vi "Teleop.vi"(0 "Call Context":T3=enum."Stop", 1 "Match Info":T2={"Autonomous Elapsed Seconds"=7.637, "TeleOp Elapsed Seconds"=2.279, "Disabled Elapsed Seconds"=0.688, "Visited Autonomous"=TRUE, "Visited TeleOp"=TRUE, "Visited Disabled"=TRUE, "Autonomous Settings"={"Autonomous Style"=enum."Independent", "VI Refnum"=refnum}}) -> ()   [LabVIEW 2018]
doc: "This VI is called for each TeleOp packet received from the DS where the robot is not disabled. It is often used to read from the joysticks and update I/O or to update setpoints for timed control loops. It should complete and return within 20 milliseconds or it may miss DS packets."
uses:
  <vilib>/Rock Robotics/WPI/DriverStation/WPI_DriverStationDerivedRobotMode.ctl
  <vilib>/Rock Robotics/WPI/DriverStation/WPI_DriverStationMatch Info.ctl
  <vilib>/Rock Robotics/WPI/ThirdParty/Phoenix-LabVIEW/Motor Controller/Controls/CTRE_Phoenix_MotorControl_MotionProfileTrajectoryPoint.ctl
  Subsystems/HatchPanel/hatchPanelNotifierCluster.ctl
  Subsystems/HatchPanel/hatchPanelEnum.ctl
  Subsystems/Cargo/cargoNotifier.ctl
  Subsystems/Cargo/cargoEnum.ctl
  Subsystems/LineAlignment/LineAlignNotifier.ctl
  Subsystems/Drive/gear notifier.ctl
  Subsystems/Climb/climbStateEnum.ctl
  Subsystems/Drive/driveCommandEnum.ctl
  Subsystems/Sensors/Limelight/LimelightPipelineMode.ctl
  Subsystems/Sensors/Limelight/LimelightModeEnum.ctl
  Subsystems/Drive/MotionProfile/Constants.vi
  <vilib>/Rock Robotics/WPI/ThirdParty/Phoenix-LabVIEW/Pigeon IMU/CTRE_PigeonIMU_TareType.ctl
panel:
  out "Output Path Points":T1[](array[typedef])
  in  "Pathname":string="L1LeftToLRF"
  # "hi there"
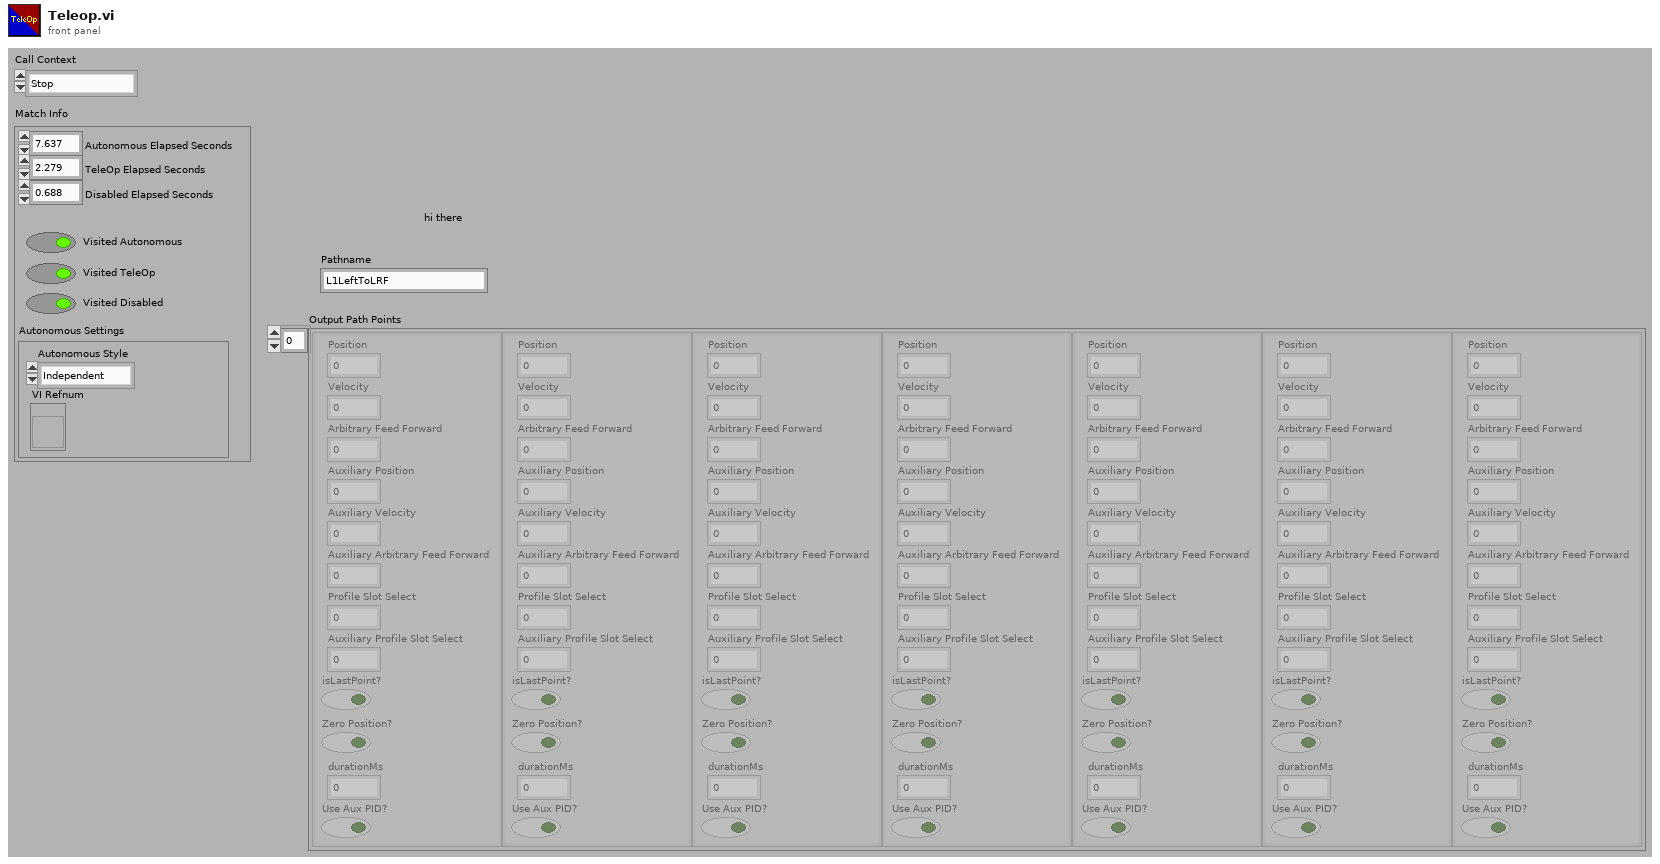
[diagram p1: front panel]
types:
  T1 = typedef "CTRE_Phoenix_MotorControl_MotionProfileTrajectoryPoint.ctl" = cluster{"Position":dbl, "Velocity":dbl, "Arbitrary Feed Forward":dbl, "Auxiliary Position":dbl, "Auxiliary Velocity":dbl, "Auxiliary Arbitrary Feed Forward":dbl, "Profile Slot Select":i32, "Auxiliary Profile Slot Select":i32, "isLastPoint?":bool, "Zero Position?":bool, "durationMs":u32, "Use Aux PID?":bool}
  T2 = typedef "WPI_DriverStationMatch Info.ctl" = cluster{"Autonomous Elapsed Seconds":dbl, "TeleOp Elapsed Seconds":dbl, "Disabled Elapsed Seconds":dbl, "Visited Autonomous":bool, "Visited TeleOp":bool, "Visited Disabled":bool, "Autonomous Settings":cluster{"Autonomous Style":enum16{"Iterative", "Independent"}, "VI Refnum":refnum<vi>}}
  T3 = typedef "WPI_DriverStationDerivedRobotMode.ctl" = enum16{"Init", "Execute", "Stop"}
  T4 = enum16{"Stach Open to Gather", "Stach Wait for Gather Extend", "Stach Gather Extended", "Stach Wait for Grab Panel", "Stach Grab Panel", "Stach Closed to Score", "Stach Wait for Sonar Signal", "Stach Wait for Score Extend", "Stach Ready to Score ", "Stach Wait for Release Panel", "Stach Release Panel", "Stach Wait for Gather Retract", "Stach Wait for Score Retract", "Stach Wait for Gather Unlock", "Stach Wait for Score Unlock", "Stach Gather End Lock", "Stach Score End Lock"}
  T5 = typedef "driveCommandEnum.ctl" = enum16{"doNothing", "Manuel", "Teleop", "Move to Target", "Climb", "Line Align", "Sonar BrakeTele", "Turn To Angle", "Auto Drive", "Test Auto Forward", "Test Auto Reversed", "Code Drive"}
  T6 = typedef "LimelightPipelineMode.ctl" = enum16{"Closest", "Leftmost", "Rightmost"}
  T7 = typedef "climbStateEnum.ctl" = enum16{"doNothing", "Auto Mode", "Safely Lower", "Test Mode"}
  T8 = typedef "gear notifier.ctl" = cluster{"High Gear?":bool, "Low Gear?":bool}
  T9 = typedef "LineAlignNotifier.ctl" = cluster{"skip 1":bool, "skip 2":bool, "LineAlign?":bool}
  T10 = typedef "cargoNotifier.ctl" = cluster{"Cargo State":T11, "Rocket?":bool, "Shoot":bool}
  T11 = typedef "cargoEnum.ctl" = enum16{"do nothing", "rocket right", "rocket left", "cargo ship left", "cargo ship right"}
  T12 = typedef "hatchPanelEnum.ctl" = enum16{"do nothing", "Stach Mode", "Climb Mode", "Retracted Closed", "Retracted Open", "Extended Closed", "Extended Open"}
  T13 = typedef "hatchPanelNotifierCluster.ctl" = cluster{"Hatch Panel State":T12, "Mechanism Motion":bool, "Gathering Claw Motion":bool, "Scoring Claw Motion":bool}
  T14 = typedef "LimelightModeEnum.ctl" = enum16{"SA - Front", "SA - Rear", "SA - Side by Side", "Vision Processing"}
  T15 = typedef "CTRE_PigeonIMU_TareType.ctl" = u8
  T16 = typedef "CTRE_PigeonIMU_DeviceRef.ctl" = cluster{"DeviceStatus":errorcluster, "Device Number":u8, "Type":T17, "Device ID":u32, "Handle":u64, "UsageFrame":u32, "Library Path":path}
  T17 = typedef "CTRE_PigeonIMU_ConnectionType.ctl" = u32
  T18 = typedef "WPI_MotorControlDeviceRef.ctl" = cluster{"DeviceStatus":errorcluster, "Type":T19, "PWM":cluster{"PWM Channel":T20, "DeadBand":T21}, "CAN":cluster{"Device Number":u8, "SetOutput VI Ref":variant, "GetOutput VI Ref":variant, "Enable VI Ref":variant, "Disable VI Ref":variant, "Data":variant}, "Invert":bool, "DIO PWM":cluster{"PWM \"Enable\" Channel":T20, "DIOChannel":T22, "PWM Rate":dbl}}
  T19 = typedef "WPI_MotorControlType.ctl" = enum16{"PWM", "CAN", "DIO PWM"}
  T20 = typedef "FPGA_DIOPWMChannel.ctl" = enum8{"PWM 0", "PWM 1", "PWM 2", "PWM 3", "PWM 4", "PWM 5", "PWM 6", "PWM 7", "PWM 8", "PWM 9", "PWM MXP 0", "PWM MXP 1", "PWM MXP 2", "PWM MXP 3", "PWM MXP 4", "PWM MXP 5", "PWM MXP 6", "PWM MXP 7", "PWM MXP 8", "PWM MXP 9", "Invalid"}
  T21 = typedef "WPI_PWMDeadband.ctl" = cluster{"Name":string, "maxPositivePwm":i32, "minPositivePwm":i32, "centerPwm":i32, "maxNegativePwm":i32, "minNegativePwm":i32, "angularRange":u16}
  T22 = typedef "FPGA_DIOChannel.ctl" = enum8{"DIO 0", "DIO 1", "DIO 2", "DIO 3", "DIO 4", "DIO 5", "DIO 6", "DIO 7", "DIO 8", "DIO 9", "DIO MXP 0", "DIO MXP 1", "DIO MXP 2", "DIO MXP 3", "DIO MXP 4", "DIO MXP 5", "DIO MXP 6", "DIO MXP 7", "DIO MXP 8", "DIO MXP 9", "DIO MXP 10", "DIO MXP 11", "DIO MXP 12", "DIO MXP 13", "DIO MXP 14", "DIO MXP 15", "SPI Port CS1", "SPI Port CS2", "SPI Port CS3", "SPI Port MISO", "SPI Port MOSI", "Invalid"}
  T23 = typedef "driveCommandEnum.ctl" = enum16{"doNothing", "Manuel", "Teleop", "Follow Path", "Move to Target", "Climb", "Line Align", "Rotate180", "LoadingStation->CargoShip", "Sonar BrakeTele", "LLCushion", "L1RightToCargo8", "Turn To Angle"}
  T24 = cluster{"Hatch Panel State":bool, "Mechanism Motion":bool, "Gathering Claw Motion":bool, "Scoring Claw Motion":bool}
  T25 = cluster{"Cargo State":bool, "Rocket?":bool, "Shoot":bool}
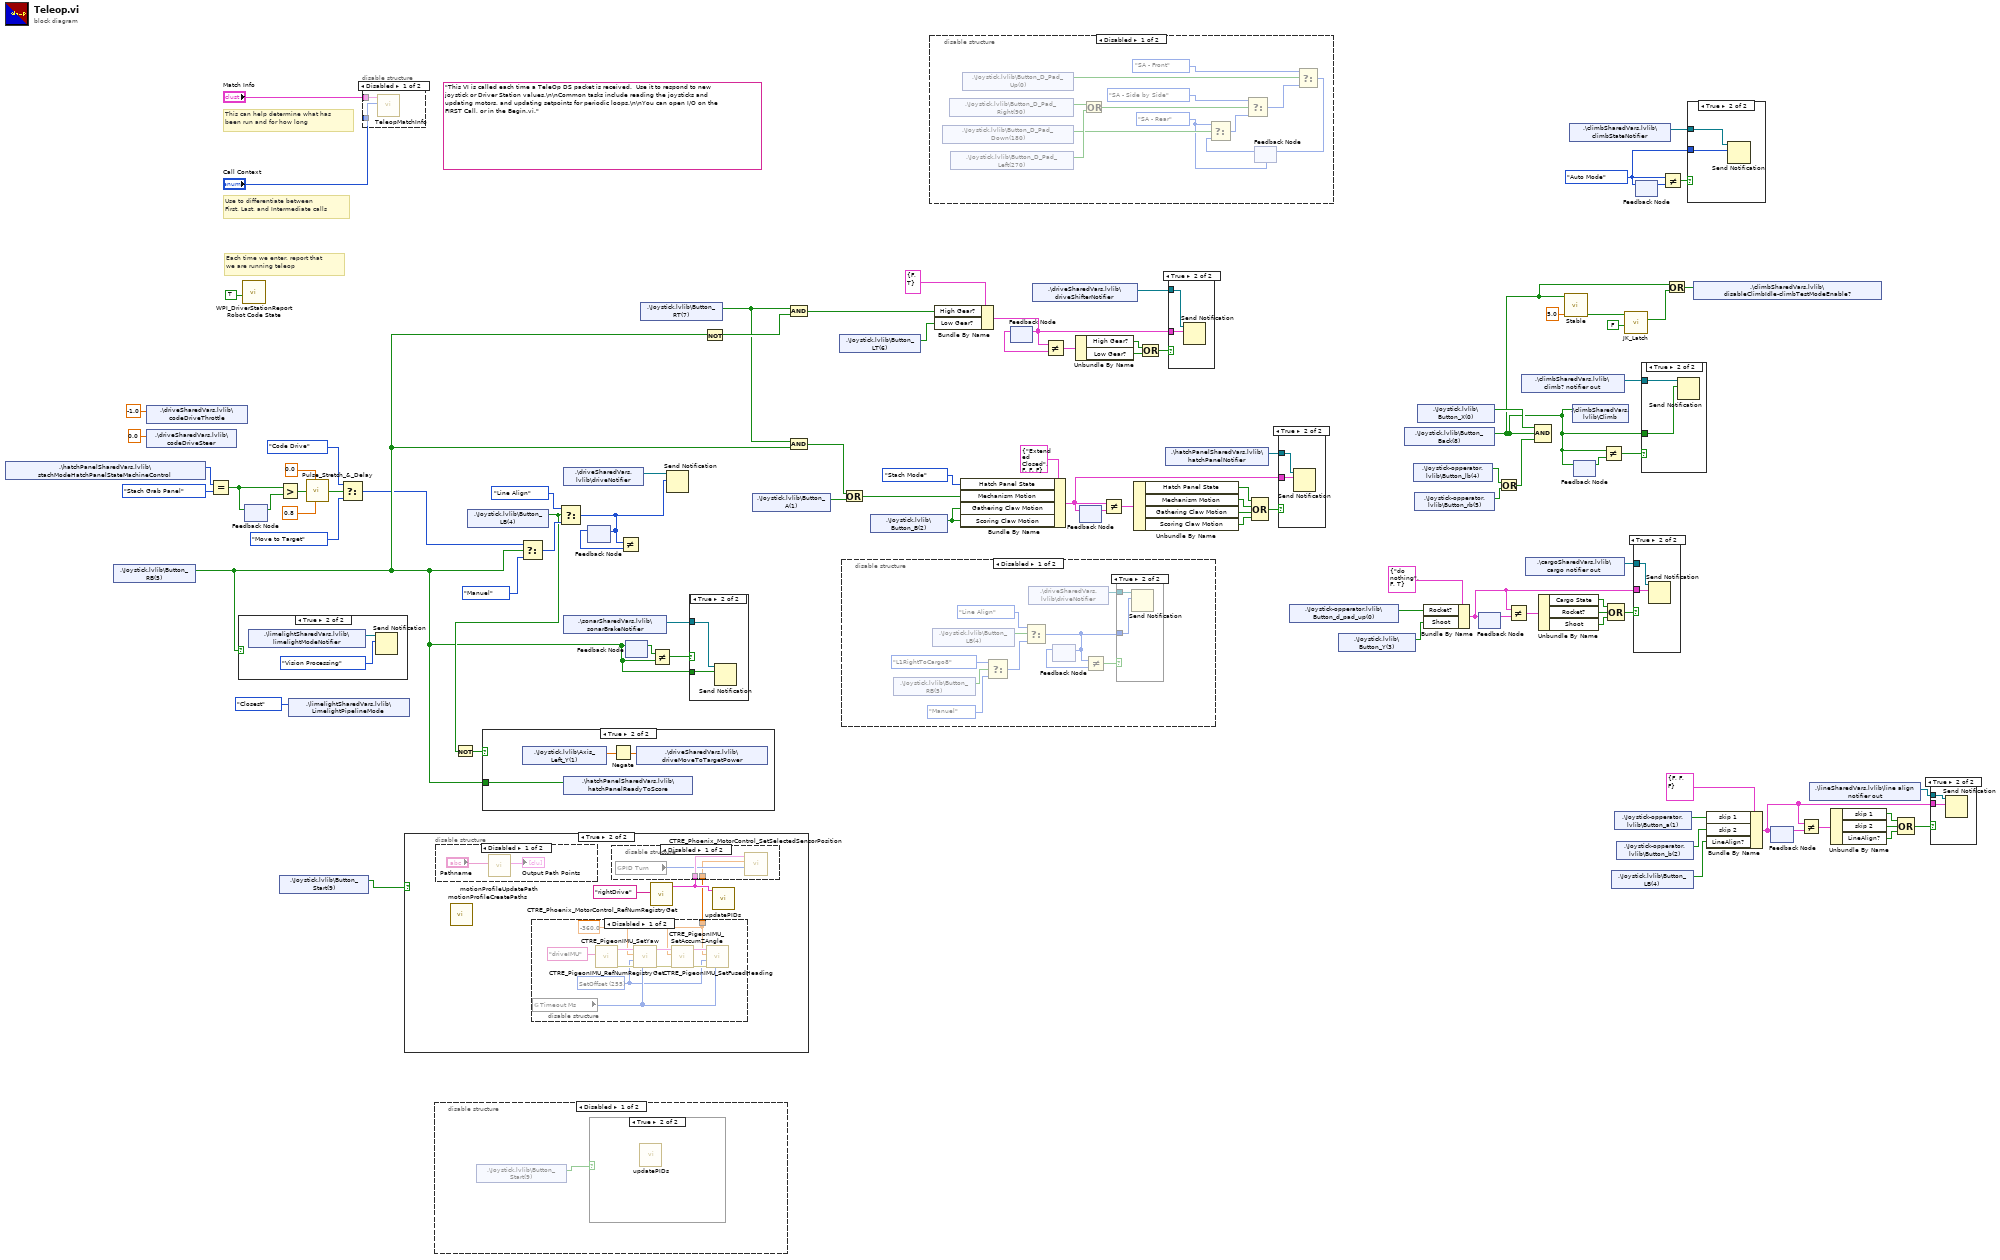
[diagram p0: block diagram]
diagram:
  w48 = climbStateEnum."Auto Mode" ("notification")
  (unwired) "This VI is called each time a TeleOp DS packet is received.  Use it to respond to new joystick or Driver Station values.\n\nCommon tasks include reading the joysticks and updating motors, and updating setpoints for periodic loops.\n\nYou can open I/O on the FIRST Call, or in the Begin.vi."
  # "Each time we enter, report that\nwe are running teleop"
  # "Use to differentiate between\nFirst, Last, and Intermediate calls"
  # "This can help determine what has\nbeen run and for how long"
  n1 = shared-variable ".\\hatchPanelSharedVars.lvlib\\stachModeHatchPanelStateMachineControl"() -> (w10:T4)  [unwired: 1 in, 1 out]
  n2 = shared-variable ".\\Joystick.lvlib\\Button_RB(5)"() -> (w21:bool)  [unwired: 1 in, 1 out]
  n3 = shared-variable ".\\driveSharedVars.lvlib\\codeDriveThrottle"(-1.0 ("codeDriveThrottle")) -> ()  [unwired: 1 in, 1 out]
  n4 = shared-variable ".\\driveSharedVars.lvlib\\codeDriveSteer"(0.0 ("codeDriveSteer")) -> ()  [unwired: 1 in, 1 out]
  n5 = Equal?(x=w10, y=T4."Stach Grab Panel") -> (x = y?=w8:bool)
  n6 = case shown="True" w21 {
    frame False {
    }
    frame True {
      n7 = shared-variable ".\\limelightSharedVars.lvlib\\limelightModeNotifier"() -> (w99:refnum<notifier>)  [unwired: 1 in, 1 out]
      n8 = Send Notification(notification=LimelightModeEnum."Vision Processing", notifier=w99) -> ()  [unwired: 1 in, 2 out]
    }
  }
  n9 = call <vilib>:"WPI_DriverStationReport Robot Code State.vi"("TeleOp"=TRUE ("Autonomous")) -> ()  [unwired: 10 in, 1 out]
  n10 = feedback #1() -> (w15:bool)  [unwired: 1 in]
  n11 = feedback-in #1(w8) -> ()
  n12 = Greater?(x=w8, y=w15) -> (0:w14:bool)
  n13 = shared-variable ".\\Joystick.lvlib\\Button_Start(9)"() -> (w33:bool)  [unwired: 1 in, 1 out]
  n14 = shared-variable ".\\limelightSharedVars.lvlib\\LimelightPipelineMode"(LimelightPipelineMode."Closest" ("LimelightPipelineMode")) -> ()  [unwired: 1 in, 1 out]
  n15 = call <userlib>:"Pulse_Stretch_&_Delay.vi"("Delay (sec)"=0.0, "In"=w14, "Width (sec)"=0.8) -> ("Out"=w11:bool)  [unwired: 2 in]
  n16 = Select(t=driveCommandEnum."Code Drive" ("notification"), s=w11, f=driveCommandEnum."Move to Target" ("notification")) -> (s? t:f=w7:T5)
  n17 = disable-structure shown="Disabled" {
    disable-tunnel: "Match Info" -> [w101 _]
    disable-tunnel: "Call Context" -> [w100 _]
    frame Disabled {
      n18 = call "TeleopMatchInfo.vi"("Call Context"=w100, "Match Info"=w101) -> ()  [unwired: 10 in]
    }
    frame Enabled {
    }
  }
  n19 = case shown="True" w33 {
    frame False {
    }
    frame True {
      n20 = disable-structure shown="Disabled" {
        frame Disabled {
          n21 = call "motionProfileUpdatePath.vi"("Pathname"="Pathname") -> ("Output Path Points"=→"Output Path Points":T1[])  [unwired: 9 in, 1 out]
        }
        frame Enabled {
        }
      }
      n22 = call "motionProfileCreatePaths.vi"() -> ()  [unwired: 12 in]
      n23 = disable-structure shown="Disabled" {
        disable-tunnel: [w110 _] -> w102
        frame Disabled {
          w110 = -360.0 ("Value")
          w111 = T15 255 items=["SetValue"=0, "AddOffset"=1, "MatchCompass"=2, "SetOffset"=255] ("TareType (SetValue)")
          n24 = global read "Constants.vi" "Timeout Ms"() -> (w116:i32)
          n25 = call <vilib>:"CTRE_PigeonIMU_RefNumRegistryGet.vi"("refnum name"="driveIMU") -> ("error out"=w118:errorcluster, "PigeonIMUDevRef"=w117:T16)  [unwired: 9 in]
          n26 = call <vilib>:"CTRE_PigeonIMU_SetYaw.vi"("timeoutMs"=w116, "error in (no error)"=w118, "TareType (SetValue)"=w111, "Value"=w110, "PigeonIMUDevRef"=w117) -> ("error out"=w115:errorcluster, "PigeonIMUDevRef"=w112:T16)  [unwired: 5 in]
          n27 = call <vilib>:"CTRE_PigeonIMU_SetAccumZAngle.vi"("error in (no error)"=w115, "Angle (Deg)"=w110, "PigeonIMUDevRef"=w112) -> ("error out"=w114:errorcluster, "PigeonIMUDevRef"=w113:T16)  [unwired: 7 in]
          n28 = call <vilib>:"CTRE_PigeonIMU_SetFusedHeading.vi"("timeoutMs"=w116, "error in (no error)"=w114, "TareType (SetValue)"=w111, "Value"=w110, "PigeonIMUDevRef 2"=w113) -> ()  [unwired: 5 in, 2 out]
        }
        frame Enabled {
        }
      }
      n29 = call <vilib>:"CTRE_Phoenix_MotorControl_RefNumRegistryGet.vi"("refnum name"="rightDrive") -> ("PhoenixMotorControlDevRef"=w103:T18)  [unwired: 9 in, 1 out]
      n30 = disable-structure shown="Disabled" {
        disable-tunnel: w103 -> [w109 _]
        disable-tunnel: w102 -> [w107 _]
        frame Disabled {
          n31 = global read "Constants.vi" "PID Turn"() -> (w108:i32)
          n32 = call <vilib>:"CTRE_Phoenix_MotorControl_SetSelectedSensorPosition.vi"("pidLoopIdx"=w108, "New Sensor Position"=w107, "PhoenixMotorControlDevRef"=w109) -> ()  [unwired: 7 in, 2 out]
        }
        frame Enabled {
        }
      }
      n33 = call "updatePIDs.vi"("MainTalon"=w103) -> ()  [unwired: 11 in]
    }
  }
  n34 = disable-structure shown="Disabled" {
    frame Disabled {
      n35 = shared-variable ".\\Joystick.lvlib\\Button_Start(9)"() -> (w120:bool)  [unwired: 1 in, 1 out]
      n36 = case shown="True" w120 {
        frame False {
        }
        frame True {
          n37 = call "updatePIDs.vi"() -> ()  [unwired: 12 in]
        }
      }
    }
    frame Enabled {
    }
  }
  n38 = shared-variable ".\\Joystick.lvlib\\Button_LB(4)"() -> (w34:bool)  [unwired: 1 in, 1 out]
  n39 = Not(x=w34) -> (.not. x?=w35:bool)
  n40 = case shown="True" w35 {
    tunnel: w21 -> [_ w121]
    frame False {
    }
    frame True {
      n41 = shared-variable ".\\Joystick.lvlib\\Axis_Left_Y(1)"() -> (w123:dbl)  [unwired: 1 in, 1 out]
      n42 = shared-variable ".\\hatchPanelSharedVars.lvlib\\hatchPanelReadyToScore"(w121) -> ()  [unwired: 1 in, 1 out]
      n43 = Negate(x=w123) -> (-x=w122:dbl)
      n44 = shared-variable ".\\driveSharedVars.lvlib\\driveMoveToTargetPower"(w122) -> ()  [unwired: 1 in, 1 out]
    }
  }
  n45 = Select(t=w7, s=w21, f=driveCommandEnum."Manuel" ("notification")) -> (s? t:f=w42:T5)
  n46 = Select(t=driveCommandEnum."Line Align" ("notification"), s=w34, f=w42) -> (s? t:f=w40:T5)
  n47 = shared-variable ".\\driveSharedVars.lvlib\\driveNotifier"() -> (w45:refnum<notifier>)  [unwired: 1 in, 1 out]
  n48 = shared-variable ".\\sonarSharedVars.lvlib\\sonarBrakeNotifier"() -> (w38:refnum<notifier>)  [unwired: 1 in, 1 out]
  n49 = feedback #2() -> (w41:T5)  [unwired: 1 in]
  n50 = feedback-in #2(w40) -> ()
  n51 = Not Equal?(x=w40, y=w41) -> ()  [unwired: 1 out]
  n52 = feedback #3() -> (w36:bool)  [unwired: 1 in]
  n53 = feedback-in #3(w21) -> ()
  n54 = shared-variable ".\\Joystick.lvlib\\Button_RT(7)"() -> (w20:bool)  [unwired: 1 in, 1 out]
  n55 = Not Equal?(x=w36, y=w21) -> (x != y?=w37:bool)
  n56 = Send Notification(notification=w40, notifier=w45) -> ()  [unwired: 1 in, 2 out]
  n57 = case shown="True" w37 {
    tunnel: w38 -> [_ w125]
    tunnel: w21 -> [_ w124]
    frame False {
    }
    frame True {
      n58 = Send Notification(notification=w124, notifier=w125) -> ()  [unwired: 1 in, 2 out]
    }
  }
  n59 = Not(x=w21) -> (.not. x?=w25:bool)
  n60 = shared-variable ".\\Joystick.lvlib\\Button_A(1)"() -> (w23:bool)  [unwired: 1 in, 1 out]
  n61 = And(x=w20, y=w25) -> (x .and. y?=w26:bool)
  n62 = And(x=w20, y=w21) -> (x .and. y?=w22:bool)
  n63 = shared-variable ".\\Joystick.lvlib\\Button_LT(6)"() -> (w82:bool)  [unwired: 1 in, 1 out]
  n64 = disable-structure shown="Disabled" {
    frame Disabled {
      n65 = shared-variable ".\\Joystick.lvlib\\Button_RB(5)"() -> (w133:bool)  [unwired: 1 in, 1 out]
      n66 = shared-variable ".\\Joystick.lvlib\\Button_LB(4)"() -> (w129:bool)  [unwired: 1 in, 1 out]
      n67 = Select(t=driveCommandEnum."L1RightToCargo8" ("notification"), s=w133, f=driveCommandEnum."Manuel" ("notification")) -> (s? t:f=w130:u16)
      n68 = Select(t=driveCommandEnum."Line Align" ("notification"), s=w129, f=w130) -> (s? t:f=w127:u16)
      n69 = shared-variable ".\\driveSharedVars.lvlib\\driveNotifier"() -> (w135:refnum<notifier>)  [unwired: 1 in, 1 out]
      n70 = feedback #4() -> (w128:u16)  [unwired: 1 in]
      n71 = feedback-in #4(w127) -> ()
      n72 = Not Equal?(x=w127, y=w128) -> (x != y?=w126:bool)
      n73 = case shown="True" w126 {
        tunnel: w135 -> [_ w137]
        tunnel: w127 -> [_ w136]
        frame False {
        }
        frame True {
          n74 = Send Notification(notification=w136, notifier=w137) -> ()  [unwired: 1 in, 2 out]
        }
      }
    }
    frame Enabled {
    }
  }
  n75 = Or(x=w22, y=w23) -> (x .or. y?=w24:bool)
  n76 = shared-variable ".\\Joystick.lvlib\\Button_B(2)"() -> (w81:bool)  [unwired: 1 in, 1 out]
  n77 = disable-structure shown="Disabled" {
    frame Disabled {
      w140 = LimelightModeEnum."SA - Rear" ("notification")
      n78 = shared-variable ".\\Joystick.lvlib\\Button_D_Pad_Down(180)"() -> (w147:bool)  [unwired: 1 in, 1 out]
      n79 = shared-variable ".\\Joystick.lvlib\\Button_D_Pad_Right(90)"() -> (w148:bool)  [unwired: 1 in, 1 out]
      n80 = shared-variable ".\\Joystick.lvlib\\Button_D_Pad_Left(270)"() -> (w149:bool)  [unwired: 1 in, 1 out]
      n81 = shared-variable ".\\Joystick.lvlib\\Button_D_Pad_Up(0)"() -> (w143:bool)  [unwired: 1 in, 1 out]
      n82 = Or(x=w148, y=w149) -> (x .or. y?=w145:bool)
      n83 = feedback #5(w140) -> (w142:T14)
      n84 = Select(t=w140, s=w147, f=w142) -> (s? t:f=w146:T14)
      n85 = Select(t=LimelightModeEnum."SA - Side by Side", s=w145, f=w146) -> (s? t:f=w144:T14)
      n86 = Select(t=LimelightModeEnum."SA - Front", s=w143, f=w144) -> (s? t:f=w141:T14)
      n87 = feedback-in #5(w141) -> ()
    }
    frame Enabled {
    }
  }
  n88 = Bundle By Name(cluster=T8 {"High Gear?"=FALSE, "Low Gear?"=TRUE} ("Cluster"), "High Gear?"=w26, "Low Gear?"=w82) -> (w51:T8)
  n89 = Bundle By Name(cluster=T13 {"Hatch Panel State"=enum."Extended Closed", "Mechanism Motion"=FALSE, "Gathering Claw Motion"=FALSE, "Scoring Claw Motion"=FALSE} ("notification"), "Hatch Panel State"=hatchPanelEnum."Stach Mode", "Mechanism Motion"=w24, "Gathering Claw Motion"=w81, "Scoring Claw Motion"=w81) -> (w57:T13)
  n90 = feedback #6() -> (w56:T8)  [unwired: 1 in]
  n91 = feedback-in #6(w51) -> ()
  n92 = shared-variable ".\\driveSharedVars.lvlib\\driveShifterNotifier"() -> (w28:refnum<notifier>)  [unwired: 1 in, 1 out]
  n93 = Not Equal?(x=w51, y=w56) -> (x != y?=w55:T8)
  n94 = Unbundle By Name(w55) -> ("High Gear?"=w54:bool, "Low Gear?"=w53:bool)
  n95 = feedback #7() -> (w64:T13)  [unwired: 1 in]
  n96 = feedback-in #7(w57) -> ()
  n97 = Not Equal?(x=w57, y=w64) -> (x != y?=w63:T24)
  n98 = Unbundle By Name(w63) -> ("Hatch Panel State"=w62:bool, "Mechanism Motion"=w61:bool, "Gathering Claw Motion"=w60:bool, "Scoring Claw Motion"=w58:bool)
  n99 = Compound Arithmetic op=OR(w54, w53) -> (w52:bool)
  n100 = shared-variable ".\\hatchPanelSharedVars.lvlib\\hatchPanelNotifier"() -> (w96:refnum<notifier>)  [unwired: 1 in, 1 out]
  n101 = case shown="True" w52 {
    tunnel: w51 -> [_ w151]
    tunnel: w28 -> [_ w150]
    frame False {
    }
    frame True {
      n102 = Send Notification(notification=w151, notifier=w150) -> ()  [unwired: 1 in, 2 out]
    }
  }
  n103 = Compound Arithmetic op=OR(w62, w61, w60, w58) -> (w59:bool)
  n104 = case shown="True" w59 {
    tunnel: w96 -> [_ w153]
    tunnel: w57 -> [_ w152]
    frame False {
    }
    frame True {
      n105 = Send Notification(notification=w152, notifier=w153) -> ()  [unwired: 1 in, 2 out]
    }
  }
  n106 = shared-variable ".\\Joystick-opperator.lvlib\\Button_d_pad_up(0)"() -> (w89:bool)  [unwired: 1 in, 1 out]
  n107 = shared-variable ".\\Joystick.lvlib\\Button_Y(3)"() -> (w86:bool)  [unwired: 1 in, 1 out]
  n108 = shared-variable ".\\Joystick.lvlib\\Button_Back(8)"() -> (w6:bool)  [unwired: 1 in, 1 out]
  n109 = shared-variable ".\\Joystick-opperator.lvlib\\Button_lb(4)"() -> (w30:bool)  [unwired: 1 in, 1 out]
  n110 = shared-variable ".\\Joystick-opperator.lvlib\\Button_rb(5)"() -> (w31:bool)  [unwired: 1 in, 1 out]
  n111 = shared-variable ".\\Joystick.lvlib\\Button_X(0)"() -> (w87:bool)  [unwired: 1 in, 1 out]
  n112 = Bundle By Name(cluster=T10 {"Cargo State"=enum."do nothing", "Rocket?"=FALSE, "Shoot"=TRUE}, "Rocket?"=w89, "Shoot"=w86) -> (w77:T10)
  n113 = feedback #8() -> (w78:T10)  [unwired: 1 in]
  n114 = feedback-in #8(w77) -> ()
  n115 = Or(x=w30, y=w31) -> (x .or. y?=w29:bool)
  n116 = Not Equal?(x=w77, y=w78) -> (x != y?=w66:T25)
  n117 = shared-variable ".\\climbSharedVars.lvlib\\climb? notifier out"() -> (w88:refnum<notifier>)  [unwired: 1 in, 1 out]
  n118 = shared-variable ".\\cargoSharedVars.lvlib\\cargo notifier out"() -> (w92:refnum<notifier>)  [unwired: 1 in, 1 out]
  n119 = Compound Arithmetic op=AND(w87, w6, w29) -> ()  [unwired: 1 out]
  n120 = Unbundle By Name(w66) -> ("Cargo State"=w69:bool, "Rocket?"=w68:bool, "Shoot"=w67:bool)
  n121 = call <userlib>:"Stable.vi"("Eval Period (sec)"=5.0, "Signal Input"=w6) -> ("Stable"=w4:bool)  [unwired: 9 in]
  n122 = shared-variable ".\\climbSharedVars.lvlib\\climbStateNotifier"() -> (w47:refnum<notifier>)  [unwired: 1 in, 1 out]
  n123 = shared-variable ".\\climbSharedVars.lvlib\\Climb"(w6) -> ()  [unwired: 1 in, 1 out]
  n124 = feedback #9() -> (w46:bool)  [unwired: 1 in]
  n125 = feedback-in #9(w6) -> ()
  n126 = Not Equal?(x=w6, y=w46) -> (x != y?=w79:bool)
  n127 = Compound Arithmetic op=OR(w69, w68, w67) -> (w65:bool)
  n128 = shared-variable ".\\Joystick.lvlib\\Button_LB(4)"() -> (w39:bool)  [unwired: 1 in, 1 out]
  n129 = shared-variable ".\\Joystick-opperator.lvlib\\Button_a(1)"() -> (w85:bool)  [unwired: 1 in, 1 out]
  n130 = shared-variable ".\\Joystick-opperator.lvlib\\Button_b(2)"() -> (w84:bool)  [unwired: 1 in, 1 out]
  n131 = call <userlib>:"JK_Latch.vi"("Reset"=FALSE, "Set"=w4) -> ("Q"=w1:bool)  [unwired: 5 in]
  n132 = case shown="True" w65 {
    tunnel: w77 -> [_ w155]
    tunnel: w92 -> [_ w154]
    frame False {
    }
    frame True {
      n133 = Send Notification(notification=w155, notifier=w154) -> ()  [unwired: 1 in, 2 out]
    }
  }
  n134 = feedback #10() -> (w50:T7)  [unwired: 1 in]
  n135 = feedback-in #10(w48) -> ()
  n136 = case shown="True" w79 {
    tunnel: w88 -> [_ w157]
    tunnel: w6 -> [_ w156]
    frame False {
    }
    frame True {
      n137 = Send Notification(notification=w156, notifier=w157) -> ()  [unwired: 1 in, 2 out]
    }
  }
  n138 = Not Equal?(x=w48, y=w50) -> (x != y?=w49:bool)
  n139 = Or(x=w6, y=w1) -> (x .or. y?=w2:bool)
  n140 = case shown="True" w49 {
    tunnel: w47 -> [_ w159]
    tunnel: w48 -> [_ w158]
    frame False {
    }
    frame True {
      n141 = Send Notification(notification=w158, notifier=w159) -> ()  [unwired: 1 in, 2 out]
    }
  }
  n142 = shared-variable ".\\climbSharedVars.lvlib\\disableClimbIdle-climbTestModeEnable?"(w2) -> ()  [unwired: 1 in, 1 out]
  n143 = Bundle By Name(cluster=T9 {"skip 1"=FALSE, "skip 2"=FALSE, "LineAlign?"=FALSE}, "skip 1"=w85, "skip 2"=w84, "LineAlign?"=w39) -> (w75:T9)
  n144 = feedback #11() -> (w76:T9)  [unwired: 1 in]
  n145 = feedback-in #11(w75) -> ()
  n146 = Not Equal?(x=w75, y=w76) -> (x != y?=w74:T9)
  n147 = shared-variable ".\\lineSharedVars.lvlib\\line align notifier out"() -> (w91:refnum<notifier>)  [unwired: 1 in, 1 out]
  n148 = Unbundle By Name(w74) -> ("skip 1"=w73:bool, "skip 2"=w72:bool, "LineAlign?"=w71:bool)
  n149 = Compound Arithmetic op=OR(w73, w72, w71) -> (w70:bool)
  n150 = case shown="True" w70 {
    tunnel: w91 -> [_ w161]
    tunnel: w75 -> [_ w160]
    frame False {
    }
    frame True {
      n151 = Send Notification(notification=w160, notifier=w161) -> ()  [unwired: 1 in, 2 out]
    }
  }
